vi "Get and Set GObj Position.vi"(8 "错误输入（无错误）":errorcluster, 9 "Mode":enum16{"Read", "Write"}(ring), 10 "位置":T1 caption="Position In", 11 "GObj Ref In":refnum<vi>) -> (0 "错误输出":errorcluster, 2 "Position":T1 caption="Position Out", 3 "GObj Ref Out":refnum<vi>)   [LabVIEW 2012, in "CtrlRef.lvlib"]
uses:
  CtrlRef.lvlib
  <vilib>/Utility/miscctls.llb/LVPositionTypeDef.ctl
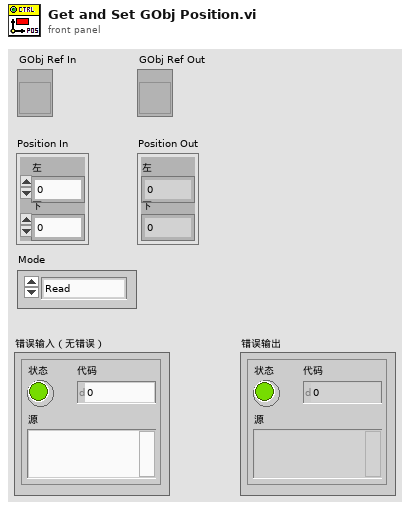
[diagram p1: front panel]
types:
  T1 = typedef "LVPositionTypeDef.ctl" = cluster{"Left":i32, "Top":i32}
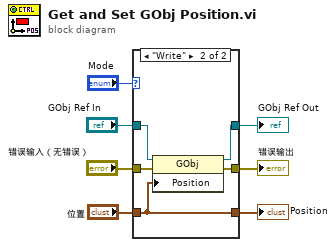
[diagram p0: block diagram]
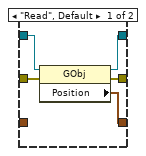
[diagram p2: hidden frame]
diagram:
  n1 = case shown="\"Write\"" "Mode" {
    tunnel: [w12 w13] -> w6
    tunnel: "错误输入（无错误）" -> [w11 w17]
    tunnel: [w10 w16] -> w4
    tunnel: "GObj Ref In" -> [w9 w15]
    tunnel: [w8 w14] -> w1
    tunnel: "位置" -> [_ w13]
    frame "Read", Default {
      n2 = property class="GObj"(reference=w9, error in=w11) -> (reference out=w8:refnum<vi>, error out=w10:errorcluster, "Position"=w12:T1)
    }
    frame "Write" {
      n3 = property class="GObj"(reference=w15, error in=w17, "Position"=w13) -> (reference out=w14:refnum<vi>, error out=w16:errorcluster)
    }
  }
  "错误输出" <- w4
  "Position" <- w6
  "GObj Ref Out" <- w1
